vi "_FPGAChannelsManager_Interface.vi"(9 "EventsIn":T1, 10 "Events":T2) -> ()   [LabVIEW 2015, in "FPGAChannelsManager.lvclass"]
uses:
  FPGAChannelsManager.lvclass
  <resource>/Framework/Providers/Veritech_GCM/Support/Framework/_Plugins/_LVCMPlugin/GCMPlugin_EventsOut.ctl
  <resource>/Framework/Providers/Veritech_GCM/Support/Framework/_Plugins/_LVCMPlugin/GCMPlugin_EventsIn.ctl
  <resource>/Framework/Providers/Veritech_GCM/Support/Framework/_Plugins/GCMPlugin/GCMPlugin.lvclass
panel:
  in  "Multicolumn Listbox":i32(listbox)
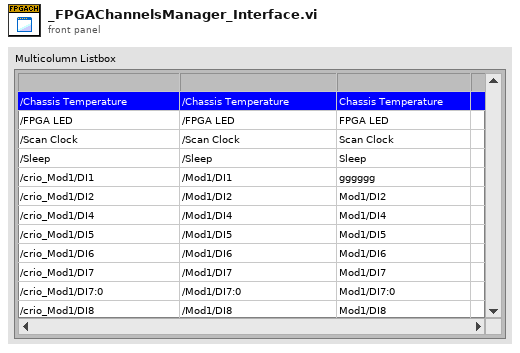
[diagram p1: front panel]
types:
  T1 = typedef "GCMPlugin.lvclass/GCMPlugin_EventsIn.ctl" = cluster{"Stop":refnum<user-event>, "ItemSelected":refnum<user-event>, "ItemDeselected":refnum<user-event>, "PluginActivated":refnum<user-event>, "PluginDeactivated":refnum<user-event>}
  T2 = typedef "GCMPlugin.lvclass/GCMPlugin_EventsOut.ctl" = cluster{"ItemEdited":refnum<user-event>}
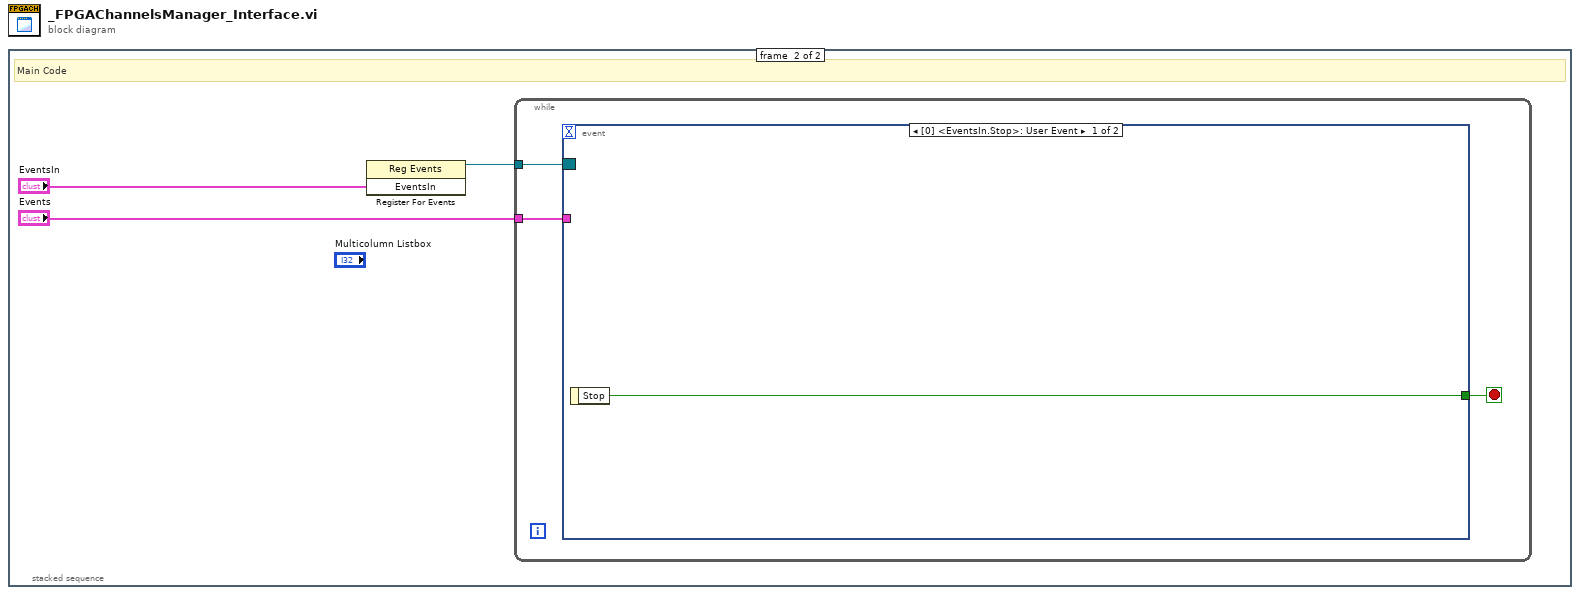
[diagram p0: block diagram]
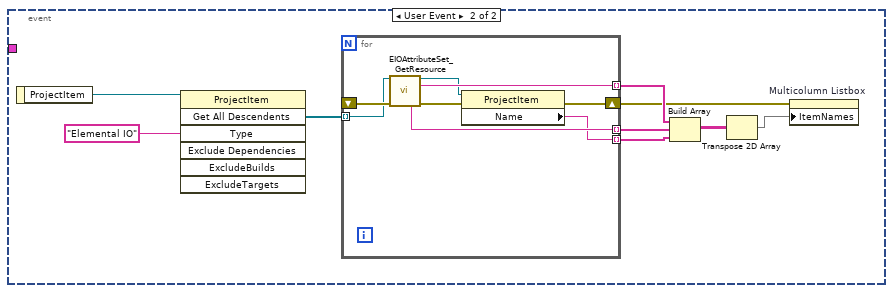
[diagram p3: hidden frame]
diagram:
  n1 = stacked-sequence {
    frame #0 {
      # "Init"
    }
    frame #1 {
      # "Main Code"
      n2 = register-events("EventsIn") -> (reference out=w2:refnum<event-registration>)  [unwired: 2 in, 1 out]
      n3 = while {
        tunnel: w2 -> [w6]
        tunnel: "Events" -> [w5]
        stop <- w4 stop-if-true
        n4 = event shown="[0] <EventsIn.Stop>: User Event" {
          selector: w6 -> [_ _]
          dyn-events: _ -> [_ _]
          timeout: _ -> [_ _]
          tunnel: w5 -> [_ _]
          tunnel: [w7 _] -> w4
          event User Event {
            n5 = event-data() -> ("Stop"=w7:bool)  [unwired: 1 in]
          }
          event User Event {
            n6 = event-data() -> ("ProjectItem"=w15:refnum<vi>)  [unwired: 1 in]
            n7 = invoke class="ProjectItem" method="Get All Descendents"(reference=w15, "Type"="Elemental IO") -> ("All Descendents"=w8:refnum<vi>[])  [unwired: 5 in, 6 out]
            n8 = for {
              tunnel: w8 -> [w22] mode=indexing
              shift-right: [w19] -> w10
              shift-left: _ -> [w24]
              tunnel: [w21] -> w14 mode=indexing
              tunnel: [w20] -> w13 mode=indexing
              tunnel: [w18] -> w9 mode=indexing
              n9 = call <resource>:"EIOAttributeSet_GetResource.vi"("EIOItem Refnum In"=w22, "error in (no error)"=w24) -> ("EIOItem Refnum Out"=w17:refnum<vi>, "resource name"=w21:string, "resource display name"=w20:string, "error out"=w23:errorcluster)  [unwired: 8 in, 2 out]
              n10 = property class="ProjectItem"(reference=w17, error in=w23) -> (error out=w19:errorcluster, "Name"=w18:string)  [unwired: 1 out]
            }
            n11 = Build Array(w14, w13, w9) -> (w12:string[][])
            n12 = Transpose 2D Array(2D array=w12) -> (transposed array=w11:string[][])
            n13 = property on="Multicolumn Listbox" class="MCListbox (strict)"(error in=w10, "ItemNames"=w11) -> ()  [unwired: 1 in, 2 out]
          }
        }
      }
    }
  }
